vi "drive commands.vi"(4 "New Command":bool, 5 "Angle Tolerance":dbl=0.02, 6 "Position":T1, 7 "Speed Setpoint":dbl, 8 "Max Wheel Speed (TPS?)":dbl=15000.0 format="%#_13g", 9 "Current Time":dbl format="%#_13g", 10 "Duration":dbl, 11 "Yaw (radians, 0=right)":dbl format="%#_13g") -> (0 "Finished":bool, 2 "Speed Right":dbl format="%#_13g", 3 "Speed Left":dbl format="%#_13g")   [LabVIEW 2015]
uses:
  Robot Global Data.vi
panel:
  in  "Ticks Per Inch":dbl=204.517
  in  "PID Turn Gains":T2={"proportional gain (Kc)"=0.6, "integral time (Ti, min)"=0.0, "derivative time (Td, min)"=0.0}
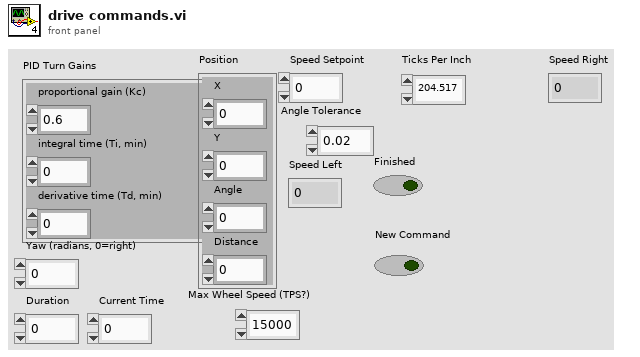
[diagram p1: front panel]
types:
  T1 = cluster{"X":dbl, "Y":dbl, "Angle":dbl, "Distance":dbl}
  T2 = cluster{"proportional gain (Kc)":dbl, "integral time (Ti, min)":dbl, "derivative time (Td, min)":dbl}
  T3 = cluster{"X":bool, "Y":bool, "Angle":bool, "Distance":bool}
  T4 = enum16{"Nothing", "Turn to Angle", "Pick Up Ball", "Drive Straight", "Drive to Target (arc)"}
  T5 = typedef "WPI_MotorControlDeviceRef.ctl" = cluster{"DeviceStatus":errorcluster, "Type":T6, "PWM":cluster{"PWM Channel":T7, "DeadBand":T8}, "CAN":cluster{"Device Number":u8, "Control Mode":T9, "Semaphore":T10, "Max Vout":dbl, "TalonSRX Control Mode":T11}, "Invert":bool}
  T6 = typedef "WPI_MotorControlType.ctl" = enum16{"PWM", "CAN", "CANTalonSRX"}
  T7 = typedef "FPGA_DIOPWMChannel.ctl" = enum8{"PWM 0", "PWM 1", "PWM 2", "PWM 3", "PWM 4", "PWM 5", "PWM 6", "PWM 7", "PWM 8", "PWM 9", "PWM MXP 0", "PWM MXP 1", "PWM MXP 2", "PWM MXP 3", "PWM MXP 4", "PWM MXP 5", "PWM MXP 6", "PWM MXP 7", "PWM MXP 8", "PWM MXP 9", "Invalid"}
  T8 = typedef "WPI_PWMDeadband.ctl" = cluster{"Name":string, "maxPositivePwm":i32, "minPositivePwm":i32, "centerPwm":i32, "maxNegativePwm":i32, "minNegativePwm":i32, "angularRange":u16}
  T9 = typedef "WPI_CANJaguar_ControlMode.ctl" = enum8{"Percent VBus", "Current", "Speed", "Position", "Voltage"}
  T10 = typedef "Semaphore RefNum" = refnum<k1>
  T11 = typedef "WPI_CANTalonSRX_APIControlMode.ctl" = enum8{"Percent VBus", "Speed", "Position", "Slave", "Unchanged / Invalid", "Voltage Compensation", "Current", "Motion Profile"}
  T12 = typedef "WPI_CANTalonSRX_GlobalStatus.ctl" = cluster{"Applied Throttle":dbl, "Module Enabled":bool, "CAN Error":errorcluster, "Closed Loop Error":dbl, "Forward Limit Switch Closed":bool, "Reverse Limit Switch Closed":bool, "Sensor Position":dbl, "Sensor Velocity":dbl, "Current":dbl, "Sticky Fault - Over Temp":bool, "Sticky Fault - Under Voltage":bool, "Sticky Fault - Forward Limit":bool, "Sticky Fault - Reverse Limit":bool, "Sticky Fault - Forward Soft Limit":bool, "Sticky Fault - Reverse Soft Limit":bool, "Brake is Enabled":bool, "Encoder Position":dbl, "Encoder Velocity":dbl, "Encoder Index Count":dbl, "Encoder A Pin State":bool, "Encoder B Pin State":bool, "Encoder Index Pin State":bool, "Analog In":dbl, "Analog In Velocity":dbl, "Temperature (C)":dbl, "Battery Voltage":dbl, "Control 5 Is Supported":bool, "Current Profile Slot Select":dbl, "Pos Div 8":bool, "Vel Div 4":bool, "Pulse Width Position":i32, "Pulse Width Velocity":i32, "Pulse Width Rise To Rise (us)":i32, "Pulse Width Rise To Fall (us)":i32, "Mot Prof Active Is Under Run":bool, "Mot Prof Active Has Under Run":bool, "Mot Prof Active Is Last":bool, "Mot Prof Active Velocity Only":bool, "Mot Prof Active Is Valid":bool, "Mot Prof Buffer Is Full":bool, "Mot Prof Active Profile Slot Select":i32, "Mot Prof NextID":i32, "Mot Prof Count":i32, "Mot Prof Active Velocity":dbl, "Mot Prof Active Position":dbl, "Mot Prof Output Enable":i32}
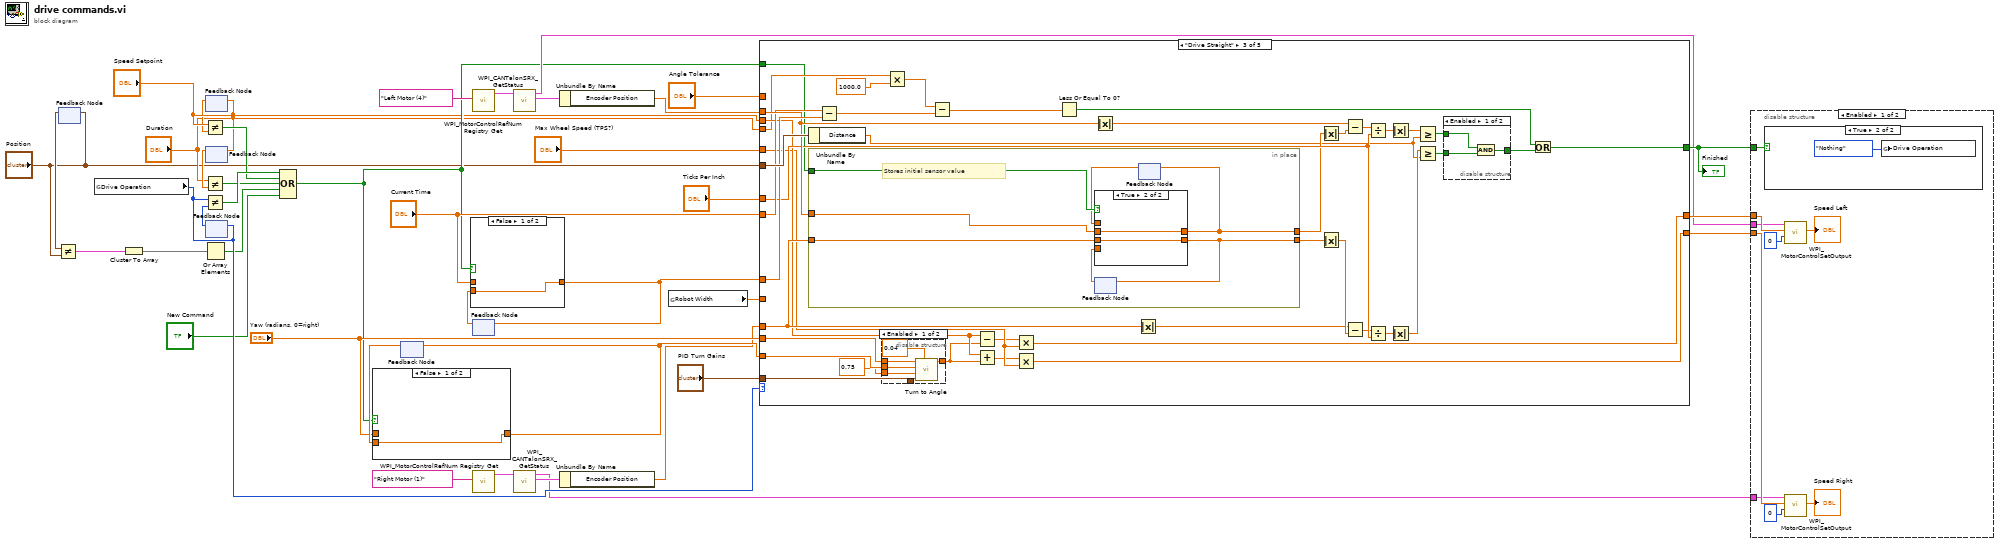
[diagram p0: block diagram]
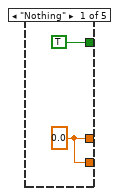
[diagram p6: hidden frame]
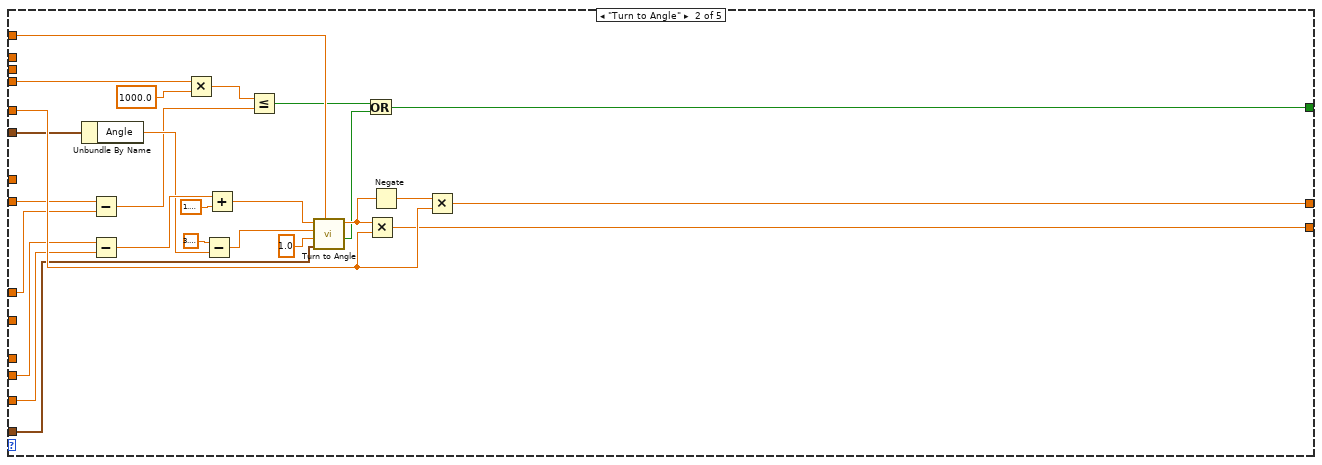
[diagram p7: hidden frame]
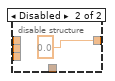
[diagram p8: hidden frame]
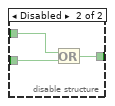
[diagram p9: hidden frame]
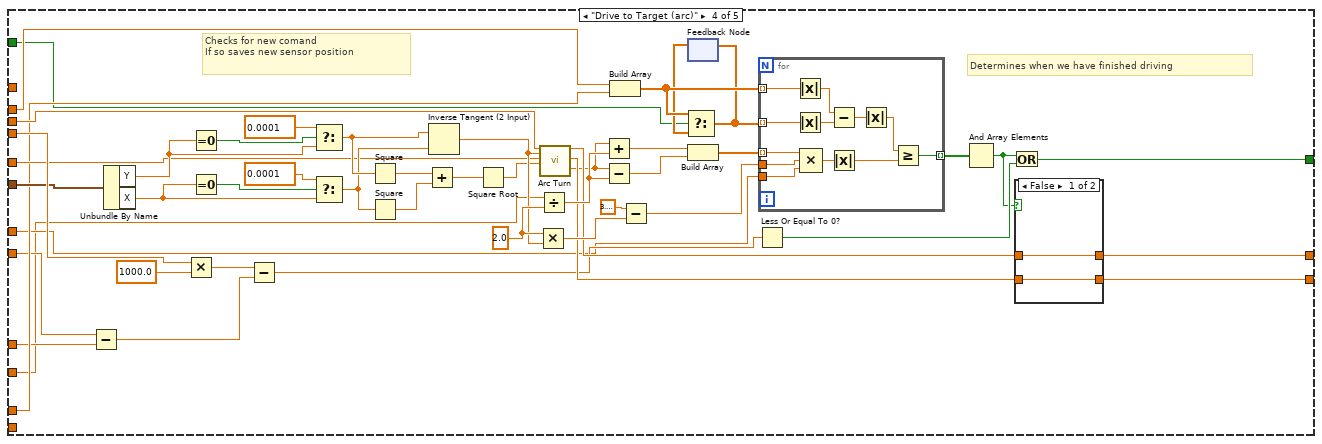
[diagram p11: hidden frame]
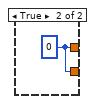
[diagram p12: hidden frame]
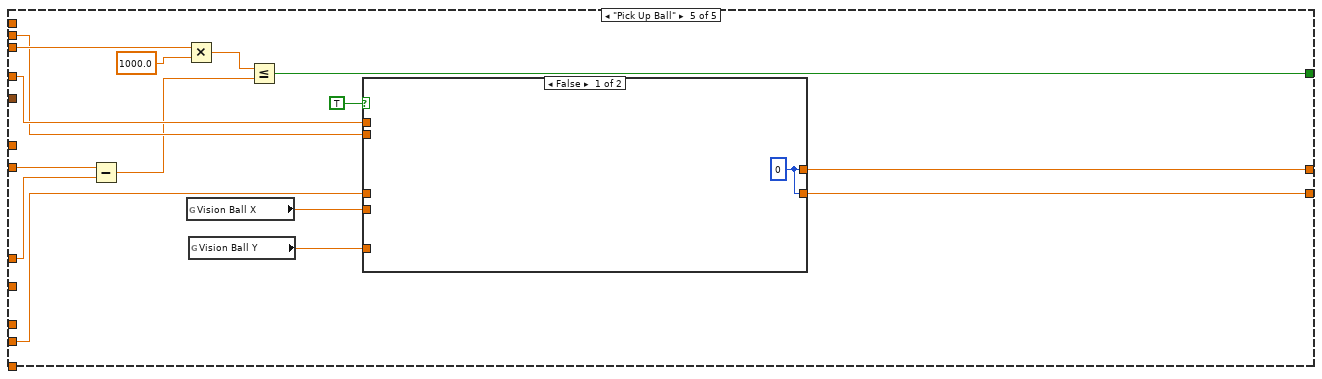
[diagram p13: hidden frame]
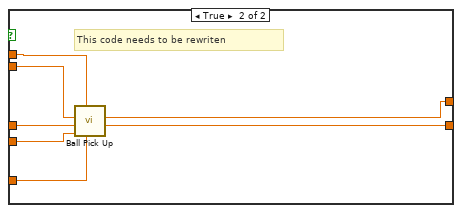
[diagram p14: hidden frame]
diagram:
  n1 = feedback #1() -> (w6:T1)  [unwired: 1 in]
  n2 = Not Equal?(x=w6, y="Position") -> (x != y?=w4:T3)
  n3 = feedback-in #1("Position") -> ()
  n4 = global read "Robot Global Data.vi" "Drive Operation"() -> (w18:T4)
  n5 = Cluster To Array(cluster=w4) -> (array=w3:bool[])
  n6 = Or Array Elements(Boolean array=w3) -> (logical OR=w2:bool)
  n7 = feedback-in #2("Speed Setpoint") -> ()
  n8 = feedback #2() -> (w11:dbl)  [unwired: 1 in]
  n9 = Not Equal?(x="Speed Setpoint", y=w11) -> (x != y?=w10:bool)
  n10 = feedback #3() -> (w9:dbl)  [unwired: 1 in]
  n11 = Not Equal?(x="Duration", y=w9) -> (x != y?=w7:bool)
  n12 = feedback-in #3("Duration") -> ()
  n13 = feedback-in #4(w18) -> ()
  n14 = feedback #4() -> (w38:T4)  [unwired: 1 in]
  n15 = Not Equal?(x=w18, y=w38) -> (x != y?=w20:bool)
  n16 = Compound Arithmetic op=OR(w20, w10, w7, w2, "New Command") -> (w13:bool)
  n17 = feedback #5() -> (w39:dbl)  [unwired: 1 in]
  n18 = case shown="False" w13 {
    tunnel: [w41 w42] -> w37
    tunnel: "Yaw (radians, 0=right)" -> [_ w42]
    tunnel: w39 -> [w41 _]
    frame False {
    }
    frame True {
      # "Saves Yaw Before Command"
    }
  }
  n19 = feedback-in #5(w37) -> ()
  n20 = call <vilib>:"WPI_MotorControlRefNum Registry Get.vi"("refnum name"="Left Motor (4)") -> ("MotorControlDevRef"=w28:T5)  [unwired: 9 in, 1 out]
  n21 = feedback #6() -> (w34:dbl)  [unwired: 1 in]
  n22 = case shown="False" w13 {
    tunnel: [w43 w44] -> w33
    tunnel: "Current Time" -> [_ w44]
    tunnel: w34 -> [w43 _]
    frame False {
    }
    frame True {
      # "Saves Time Before Command"
    }
  }
  n23 = feedback-in #6(w33) -> ()
  n24 = call <vilib>:"WPI_MotorControlRefNum Registry Get.vi"("refnum name"="Right Motor (1)") -> ("MotorControlDevRef"=w29:T5)  [unwired: 9 in, 1 out]
  n25 = call <vilib>:"WPI_CANTalonSRX_GetStatus.vi"("CAN Talon SRX Ref"=w28) -> ("Talon SRX Status"=w24:T12, "CAN Talon SRX Ref"=w14:T5)  [unwired: 8 in, 1 out]
  n26 = call <vilib>:"WPI_CANTalonSRX_GetStatus.vi"("CAN Talon SRX Ref"=w29) -> ("Talon SRX Status"=w25:T12, "CAN Talon SRX Ref"=w15:T5)  [unwired: 8 in, 1 out]
  n27 = Unbundle By Name(w24) -> ("Encoder Position"=w23:dbl)
  n28 = Unbundle By Name(w25) -> ("Encoder Position"=w22:dbl)
  n29 = global read "Robot Global Data.vi" "Robot Width"() -> (w19:dbl)
  n30 = case shown="\"Drive Straight\"" w18 {
    tunnel: [TRUE w48 w76 w169 w202] -> w17
    tunnel: [w46 w69 w75 w155 w213] -> w16
    tunnel: [w46 w68 w74 w156 w212] -> w30
    tunnel: "Duration" -> [_ w71 w103 w181 w214]
    tunnel: "Position" -> [_ w63 w113 w172 _]
    tunnel: "Yaw (radians, 0=right)" -> [_ w67 w107 _ w210]
    tunnel: "Max Wheel Speed (TPS?)" -> [_ w70 w102 w152 w211]
    tunnel: "Speed Setpoint" -> [_ _ w104 w153 w209]
    tunnel: w37 -> [_ w66 w108 _ _]
    tunnel: "PID Turn Gains" -> [_ w59 w111 _ _]
    tunnel: w33 -> [_ w49 w112 w143 w205]
    tunnel: "Current Time" -> [_ w50 w106 w144 w204]
    tunnel: "Angle Tolerance" -> [_ w53 _ _ _]
    tunnel: w23 -> [_ _ w110 w147 _]
    tunnel: w22 -> [_ _ w109 w146 _]
    tunnel: "Ticks Per Inch" -> [_ _ w105 w139 _]
    tunnel: w13 -> [_ _ w77 w145 _]
    tunnel: w19 -> [_ _ _ w138 _]
    frame "Nothing" {
      w46 = 0.0
    }
    frame "Turn to Angle" {
      n31 = Unbundle By Name(w63) -> ("Angle"=w62:dbl)
      n32 = Subtract(x=w50, y=w49) -> (x-y=w52:dbl)
      n33 = Subtract(x=w67, y=w66) -> (x-y=w65:dbl)
      n34 = Multiply(x=w71, y=1000.0) -> (x*y=w51:dbl)
      n35 = Subtract(x=3.141592653589793, y=w62) -> (x-y=w56:dbl)
      n36 = Add(x=w65, y=1.5707963267948966) -> (x+y=w57:dbl)
      n37 = Less Or Equal?(x=w51, y=w52) -> (x <= y?=w47:bool)
      n38 = call "Turn to Angle.vi"("Angle Tolerance"=w53, "PID Gains"=w59, "Rotation Multiplier"=1.0, "Target angle"=w56, "Angle (radians; 0 = right)"=w57) -> ("Finished?"=w54:bool, "Turn Set Point"=w55:dbl)  [unwired: 2 in]
      n39 = Or(x=w47, y=w54) -> (x .or. y?=w48:bool)
      n40 = Multiply(x=w55, y=w70) -> (x*y=w69:dbl)
      n41 = Negate(x=w55) -> (-x=w60:dbl)
      n42 = Multiply(x=w60, y=w70) -> (x*y=w68:dbl)
    }
    frame "Drive Straight" {
      n43 = Unbundle By Name(w113) -> ("Distance"=w82:dbl)
      n44 = in-place {
        in-place-border: w77 -> [w133]
        in-place-border: w110 -> [w127]
        in-place-border: w109 -> [w132]
        in-place-border: [w131] -> w95
        in-place-border: [w128] -> w94
        # "Stores initial sensor value"
        n45 = feedback #7() -> (w130:dbl)  [unwired: 1 in]
        n46 = feedback #8() -> (w129:dbl)  [unwired: 1 in]
        n47 = case shown="True" w133 {
          tunnel: [w135 w137] -> w131
          tunnel: w127 -> [_ w137]
          tunnel: w129 -> [w135 _]
          tunnel: [w134 w136] -> w128
          tunnel: w132 -> [_ w136]
          tunnel: w130 -> [w134 _]
          frame False {
          }
          frame True {
          }
        }
        n48 = feedback-in #7(w128) -> ()
        n49 = feedback-in #8(w131) -> ()
      }
      n50 = Subtract(x=w106, y=w112) -> (x-y=w101:dbl)
      n51 = disable-structure shown="Enabled" {
        disable-tunnel: w111 -> [w119 _]
        disable-tunnel: w108 -> [w118 _]
        disable-tunnel: w107 -> [w117 _]
        disable-tunnel: [w115 0.0] -> w73
        disable-tunnel: 0.75 ("Rotation Multiplier") -> [w114 _]
        frame Enabled {
          n52 = call "Turn to Angle.vi"("Angle Tolerance"=0.04, "PID Gains"=w119, "Rotation Multiplier"=w114, "Target angle"=w118, "Angle (radians; 0 = right)"=w117) -> ("Turn Set Point"=w115:dbl)  [unwired: 2 in, 1 out]
        }
        frame Disabled {
        }
      }
      n53 = Multiply(x=w103, y=1000.0) -> (x*y=w99:dbl)
      n54 = Subtract(x=w99, y=w101) -> (x-y=w98:dbl)
      n55 = Subtract(x=w104, y=w73) -> (x-y=w97:dbl)
      n56 = Add(x=w104, y=w73) -> (x+y=w96:dbl)
      n57 = Multiply(x=w97, y=w102) -> (x*y=w74:dbl)
      n58 = Multiply(x=w96, y=w102) -> (x*y=w75:dbl)
      n59 = Less Or Equal To 0?(x=w98) -> (x <= 0?=w83:bool)
      n60 = Absolute Value(x=w110) -> (abs(x)=w89:dbl)
      n61 = Absolute Value(x=w109) -> (abs(x)=w87:dbl)
      n62 = Absolute Value(x=w95) -> (abs(x)=w90:dbl)
      n63 = Absolute Value(x=w94) -> (abs(x)=w88:dbl)
      n64 = Subtract(x=w89, y=w90) -> (x-y=w93:dbl)
      n65 = Subtract(x=w87, y=w88) -> (x-y=w92:dbl)
      n66 = Divide(x=w93, y=w105) -> (x/y=w91:dbl)
      n67 = Divide(x=w92, y=w105) -> (x/y=w86:dbl)
      n68 = Absolute Value(x=w91) -> (abs(x)=w84:dbl)
      n69 = Absolute Value(x=w86) -> (abs(x)=w85:dbl)
      n70 = Greater Or Equal?(x=w84, y=w82) -> (x >= y?=w81:bool)
      n71 = Greater Or Equal?(x=w85, y=w82) -> (x >= y?=w80:bool)
      n72 = disable-structure shown="Enabled" {
        disable-tunnel: w81 -> [w123 w126]
        disable-tunnel: w80 -> [w122 w125]
        disable-tunnel: [w121 w124] -> w79
        frame Enabled {
          n73 = And(x=w123, y=w122) -> (x .and. y?=w121:bool)
        }
        frame Disabled {
          n74 = Or(x=w126, y=w125) -> (x .or. y?=w124:bool)
        }
      }
      n75 = Or(x=w83, y=w79) -> (x .or. y?=w76:bool)
    }
    frame "Drive to Target (arc)" {
      w177 = 2.0 ("x")
      # "Checks for new comand\nIf so saves new sensor position"
      # "Determines when we have finished driving"
      n76 = Subtract(x=w144, y=w143) -> (x-y=w142:dbl)
      n77 = Unbundle By Name(w172) -> ("Y"=w158:dbl, "X"=w159:dbl)
      n78 = Multiply(x=w181, y=1000.0) -> (x*y=w141:dbl)
      n79 = Equal To 0?(x=w158) -> (x = 0?=w162:bool)
      n80 = Equal To 0?(x=w159) -> (x = 0?=w164:bool)
      n81 = Subtract(x=w141, y=w142) -> (x-y=w140:dbl)
      n82 = Select(t=0.0001, s=w162, f=w158) -> (s? t:f=w161:dbl)
      n83 = Select(t=0.0001, s=w164, f=w159) -> (s? t:f=w160:dbl)
      n84 = Square(x=w161) -> (x^2=w183:dbl)
      n85 = Square(x=w160) -> (x^2=w185:dbl)
      n86 = Add(x=w183, y=w185) -> (x+y=w184:dbl)
      n87 = Inverse Tangent (2 Input)(1:w160, 2:w161) -> (0:w154:dbl)
      n88 = Square Root(x=w184) -> (sqrt(x)=w151:dbl)
      n89 = Multiply(x=w177, y=w154) -> (x*y=w179:dbl)
      n90 = Divide(x=w138, y=w177) -> (x/y=w176:dbl)
      n91 = call "Arc Turn.vi"("Speed Setpoint (0-1)"=w153, "Angle Radians (0 = Right)"=w154, "Max Speed (TPS)"=w152, "Distance"=w151) -> ("Left Speed"=w150:dbl, "Right Speed"=w149:dbl, "Radius"=w148:dbl)  [unwired: 13 in]
      n92 = Add(x=w148, y=w176) -> (x+y=w175:dbl)
      n93 = Subtract(x=w148, y=w176) -> (x-y=w174:dbl)
      n94 = Build Array(w147, w146) -> (w167:dbl[])
      n95 = Subtract(x=3.141592653589793, y=w179) -> (x-y=w178:dbl)
      n96 = feedback #9() -> (w166:dbl[])  [unwired: 1 in]
      n97 = Select(t=w167, s=w145, f=w166) -> (s? t:f=w165:dbl[])
      n98 = feedback-in #9(w165) -> ()
      n99 = Build Array(w175, w174) -> (w173:dbl[])
      n100 = Less Or Equal To 0?(x=w140) -> (x <= 0?=w170:bool)
      n101 = for {
        tunnel: w178 -> [w195]
        tunnel: w173 -> [w196] mode=indexing
        tunnel: w167 -> [w190] mode=indexing
        tunnel: w165 -> [w200] mode=indexing
        tunnel: [w198] -> w171 mode=indexing
        tunnel: w139 -> [w189]
        n102 = Absolute Value(x=w190) -> (abs(x)=w192:dbl)
        n103 = Absolute Value(x=w200) -> (abs(x)=w191:dbl)
        n104 = Compound Arithmetic op=MULTIPLY(w196, w195, w189) -> (w194:dbl)
        n105 = Subtract(x=w192, y=w191) -> (x-y=w199:dbl)
        n106 = Absolute Value(x=w194) -> (abs(x)=w197:dbl)
        n107 = Absolute Value(x=w199) -> (abs(x)=w193:dbl)
        n108 = Greater Or Equal?(x=w193, y=w197) -> (x >= y?=w198:bool)
      }
      n109 = And Array Elements(Boolean array=w171) -> (logical AND=w168:bool)
      n110 = Or(x=w168, y=w170) -> (x .or. y?=w169:bool)
      n111 = case shown="False" w168 {
        tunnel: [w186 w188] -> w155
        tunnel: [w187 w188] -> w156
        tunnel: w150 -> [w187 _]
        tunnel: w149 -> [w186 _]
        frame False {
        }
        frame True {
          w188 = 0
        }
      }
    }
    frame "Pick Up Ball" {
      n112 = Subtract(x=w204, y=w205) -> (x-y=w203:dbl)
      n113 = Multiply(x=w214, y=1000.0) -> (x*y=w206:dbl)
      n114 = global read "Robot Global Data.vi" "Vision Ball X"() -> (w208:dbl)
      n115 = global read "Robot Global Data.vi" "Vision Ball Y"() -> (w207:dbl)
      n116 = Less Or Equal?(x=w206, y=w203) -> (x <= y?=w202:bool)
      n117 = case shown="False" TRUE {
        tunnel: [w216 w219] -> w213
        tunnel: [w216 w220] -> w212
        tunnel: w211 -> [_ w223]
        tunnel: w210 -> [_ w221]
        tunnel: w209 -> [_ w222]
        tunnel: w208 -> [_ w218]
        tunnel: w207 -> [_ w217]
        frame False {
          w216 = 0
        }
        frame True {
          # "This code needs to be rewriten"
          n118 = call "Ball Pick Up.vi"("Ball Y"=w217, "Max Speed"=w223, "Ball X"=w218, "Yaw"=w221, "Speed Setpoint"=w222) -> ("Speed Right"=w219:dbl, "Speed Left"=w220:dbl)  [unwired: 5 in]
        }
      }
    }
  }
  "Finished" <- w17
  n119 = disable-structure shown="Enabled" {
    disable-tunnel: w30 -> [w232 _]
    disable-tunnel: w17 -> [w231 _]
    disable-tunnel: w16 -> [w229 _]
    disable-tunnel: w15 -> [w227 _]
    disable-tunnel: w14 -> [w226 _]
    frame Enabled {
      n120 = case shown="True" w231 {
        frame False {
        }
        frame True {
          n121 = global write "Robot Global Data.vi" "Drive Operation"(T4."Nothing" ("Drive Operation")) -> ()
        }
      }
      n122 = call <vilib>:"WPI_MotorControlSetOutput.vi"("Sync Group / Parameter Slot"=u8 0, "Output"=w232, "MotorControlDevRef"=w226) -> ("Motor Output"=→"Speed Left":dbl)  [unwired: 6 in, 2 out]
      n123 = call <vilib>:"WPI_MotorControlSetOutput.vi"("Sync Group / Parameter Slot"=u8 0, "Output"=w229, "MotorControlDevRef"=w227) -> ("Motor Output"=→"Speed Right":dbl)  [unwired: 6 in, 2 out]
    }
    frame Disabled {
    }
  }
